vi "AlliGator Add Missing Parameter Map Parameters.vi"(8 "Error In":errorcluster, 9 "Parameter_Flattened_Map in":dbl[][](array[numeric]), 11 "Parameter Names":string[](array[string])) -> (0 "Error Out":errorcluster, 1 "Parameter_Flattened_Map out":dbl[][](array[numeric]), 3 "[Decay Fit Parameter Name] out":T1[](array[typedef]))   [LabVIEW 2021, in "AlliGator Python Plugins.lvlib"]
doc: "Complements python function output parameter map by adding \"NaN\" instead of the missing parameters.\n\nThe map needs to be complete to be displayable in AlliGator, even though the python function might only ouput a few parameters."
uses:
  AlliGator Python Plugins.lvlib
  Fits/IRF(X)PSED/Decay Fit Parameters & Derived Quantities List.ctl
  ec1117ef-afb6-46a0-baf7-935b1c1180a5.vi
  Fits/Fits.lvlib
panel:
  # "see the AlliGator License on the block diagram (Ctrl+E or Window:Show Block Diagram)"
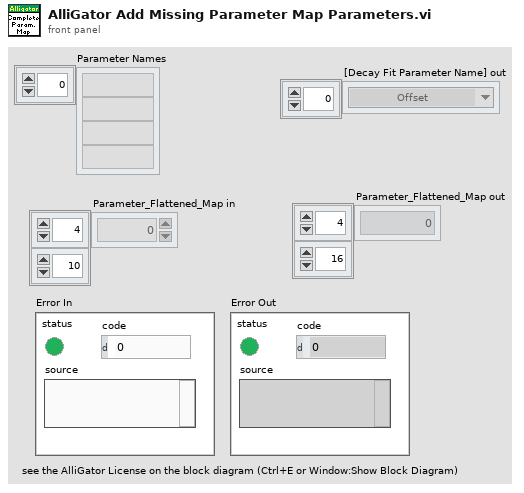
[diagram p1: front panel]
types:
  T1 = typedef "Fits.lvlib/Decay Fit Parameters & Derived Quantities List.ctl" = enum16{"Offset", "Baseline", "A_1", "tau_1", "A_2", "tau_2", "<tau>_a", "f1_a", "f2_a", "<tau>_i", "f1_i", "f2_i", "-", "R^2", "Chi^2"}
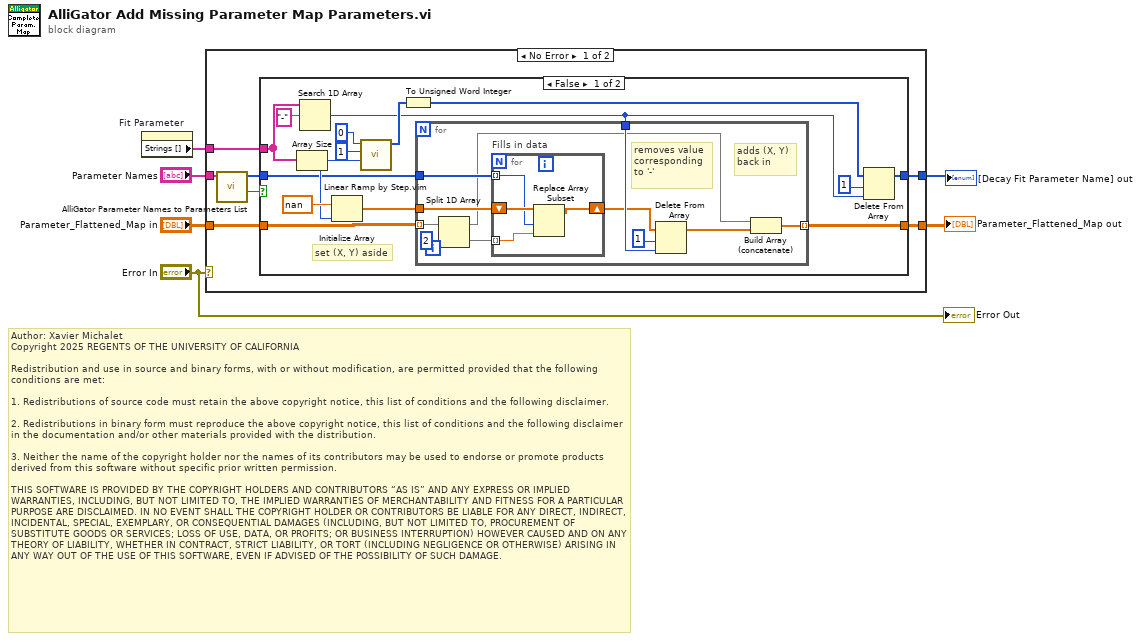
[diagram p0: block diagram]
diagram:
  # "Author: Xavier Michalet\nCopyright 2025 REGENTS OF THE UNIVERSITY OF CALIFORNIA\n\nRedistribution and use in source and binary forms, with or without modification, are permitted provided that the following conditions are met:\n\n1. Redistributions of source code must retain the above copyright notice, this list of conditions and the following disclaimer.\n\n2. Redistributions in binary form must reproduce the above copyright notice, this list of conditions and the following disclaimer in the documentation and/or other materials provided with the distribution.\n\n3. Neither the name of the copyright holder nor the names of its contributors may be used to endorse or promote products derived from this software without specific prior written permission.\n\nTHIS SOFTWARE IS PROVIDED BY THE COPYRIGHT HOLDERS AND CONTRIBUTORS “AS IS” AND ANY EXPRESS OR IMPLIED WARRANTIES, INCLUDING, BUT NOT LIMITED TO, THE IMPLIED WARRANTIES OF MERCHANTABILITY AND FITNESS FOR A PARTICULAR PURPOSE ARE DISCLAIMED. IN NO EVENT SHALL THE COPYRIGHT HOLDER OR CONTRIBUTORS BE LIABLE FOR ANY DIRECT, INDIRECT, INCIDENTAL, SPECIAL, EXEMPLARY, OR CONSEQUENTIAL DAMAGES (INCLUDING, BUT NOT LIMITED TO, PROCUREMENT OF SUBSTITUTE GOODS OR SERVICES; LOSS OF USE, DATA, OR PROFITS; OR BUSINESS INTERRUPTION) HOWEVER CAUSED AND ON ANY THEORY OF LIABILITY, WHETHER IN CONTRACT, STRICT LIABILITY, OR TORT (INCLUDING NEGLIGENCE OR OTHERWISE) ARISING IN ANY WAY OUT OF THE USE OF THIS SOFTWARE, EVEN IF ADVISED OF THE POSSIBILITY OF SUCH DAMAGE."
  n1 = property on="Fit Parameter" class="Enum (strict)"() -> ("Strings []"=w1:string[])  [unwired: 2 in, 2 out]
  n2 = case shown="No Error" "Error In" {
    tunnel: "Parameter Names" -> [w13 _]
    tunnel: [w10 _] -> w5
    tunnel: "Parameter_Flattened_Map in" -> [w9 _]
    tunnel: [w8 _] -> w3
    tunnel: w1 -> [w7 _]
    frame No Error {
      n3 = call "AlliGator Parameter Names to Parameters List.vi"("Parameter Names"=w13) -> ("Complete Map"=w12:bool, "[Decay Fit Parameter Name]"=w11:T1[])  [unwired: 9 in]
      n4 = case shown="False" w12 {
        tunnel: w11 -> [w14 w45]
        tunnel: [w20 w45] -> w10
        tunnel: w9 -> [w28 w44]
        tunnel: [w24 w44] -> w8
        tunnel: w7 -> [w22 _]
        frame False {
          # "set (X, Y) aside"
          n5 = Array Size(array=w22) -> (size(s)=w16:i32)
          n6 = Search 1D Array(1D array=w22, element="-") -> (index of element=w19:i32)  [unwired: 1 in]
          n7 = Initialize Array(nan ("new element/subarray"), w16) -> (w15:dbl[])
          n8 = call "Linear Ramp by Step.vim"("# Elements (1)"=w16, "Step (1)"=u16 1, "Start (0)"=u16 0) -> ("Ramp"=w26:i32[])  [unwired: 8 in]
          n9 = To Unsigned Word Integer(number=w26) -> (unsigned 16bit integer=w23:u16[])
          n10 = for {
            tunnel: w28 -> [w39] mode=indexing
            tunnel: [w30] -> w24 mode=indexing
            tunnel: w19 -> [w37]
            tunnel: w15 -> [w35]
            tunnel: w14 -> [w34]
            # "adds (X, Y) back in"
            # "removes value\ncorresponding\nto '-'"
            n11 = Split 1D Array(array=w39, index=2) -> (first subarray=w29:dbl[], second subarray=w32:dbl[])
            n12 = for "Fills in data" {
              tunnel: w32 -> [w41] mode=indexing
              tunnel: w34 -> [w42] mode=indexing
              shift-right: [w40] -> w33
              shift-left: w35 -> [w43]
              n13 = Replace Array Subset(array=w43, new element=w41, index=w42) -> (w40:dbl[])
            }
            n14 = Delete From Array(array=w33, length=1, index=w37) -> (array with subset deleted=w38:dbl[])  [unwired: 1 out]
            n15 = Build Array (concatenate)(w29, w38) -> (w30:dbl[])
          }
          n16 = Delete From Array(array=w23, length=1, index=w19) -> (array with subset deleted=w20:u16[])  [unwired: 1 out]
        }
        frame True {
        }
      }
    }
    frame Error {
    }
  }
  "Parameter_Flattened_Map out" <- w3
  "[Decay Fit Parameter Name] out" <- w5
  "Error Out" <- "Error In"
